vi "Write Logged Data.vi"(8 "error in (no error)":errorcluster, 10 "Data":T1[](array[typedef]), 11 "Logger Interface in":refnum<class "Logger Interface.lvclass">) -> (0 "error out":errorcluster, 3 "Logger Interface out":refnum<class "Logger Interface.lvclass">)   [LabVIEW 2020, in "Frame Logging.lvlib" / "Logger Interface.lvclass"]
uses:
  Logger Interface.lvclass
  Shared/Frame.ctl
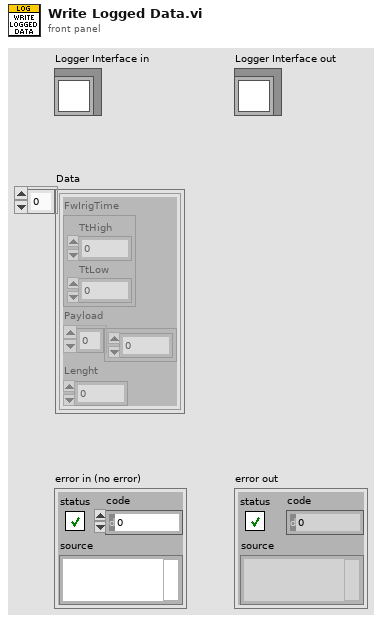
[diagram p1: front panel]
types:
  T1 = typedef "Frame.ctl" = cluster{"FwIrigTime":cluster{"TtHigh":u32, "TtLow":u32}, "Payload":u8[], "Lenght":u32}
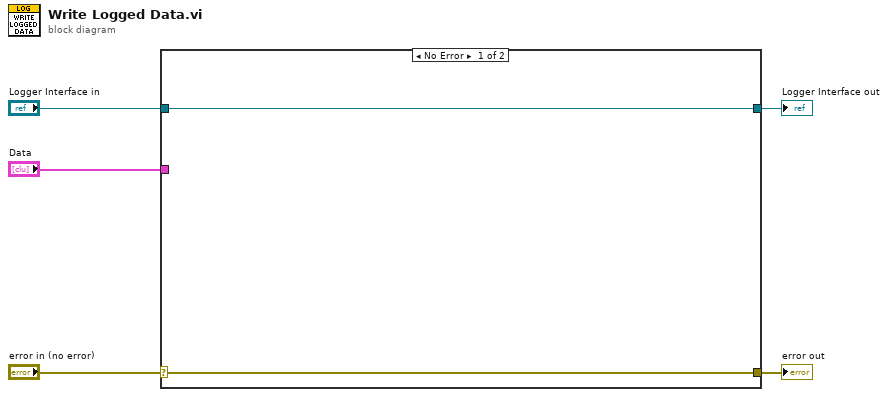
[diagram p0: block diagram]
diagram:
  n1 = case shown="No Error" "error in (no error)" {
    selector: "error in (no error)" -> [w6 w9]
    tunnel: [w6 w9] -> w4
    tunnel: [w7 w8] -> w2
    tunnel: "Logger Interface in" -> [w7 w8]
    tunnel: "Data" -> [_ _]
    frame No Error {
    }
    frame Error {
    }
  }
  "error out" <- w4
  "Logger Interface out" <- w2
